vi "Save Data.vi"(8 "error in (no error)":errorcluster, 10 "signal out":waveform(dbl), 11 "Txt in":refnum<class "Txt.lvclass">) -> (0 "error out":errorcluster, 3 "Txt out":refnum<class "Txt.lvclass">)   [LabVIEW 2020, in "Txt.lvlib" / "Txt.lvclass"]
uses:
  Txt.lvclass
  Txt.lvclass/Txt.ctl
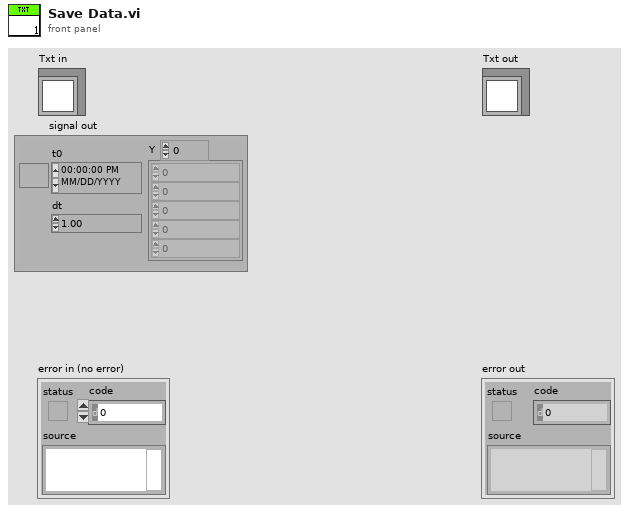
[diagram p1: front panel]
types:
  T1 = enum16{"open", "replace", "create", "open or create", "replace or create", "replace or create with confirmation"}
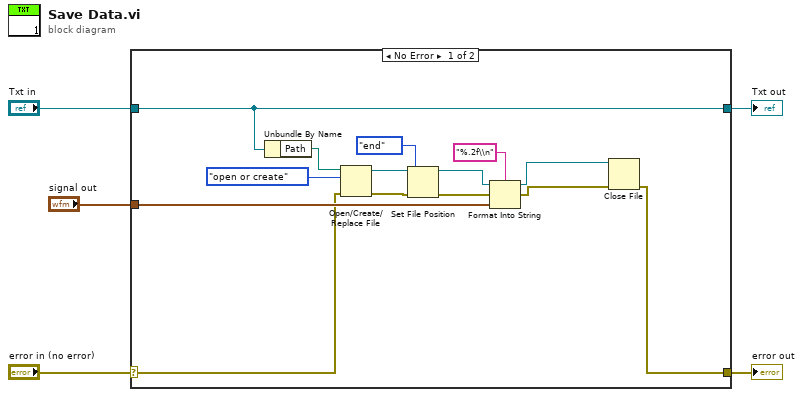
[diagram p0: block diagram]
diagram:
  n1 = case shown="No Error" "error in (no error)" {
    selector: "error in (no error)" -> [w7 w21]
    tunnel: [w6 w21] -> w4
    tunnel: [w9 w20] -> w2
    tunnel: "Txt in" -> [w9 w20]
    tunnel: "signal out" -> [w8 _]
    frame No Error {
      n2 = Unbundle By Name(w9) -> ("Path"=w19:path)
      n3 = Open/Create/Replace File(file path (use dialog)=w19, error in=w7, operation (0:open)=T1."open or create") -> (refnum out=w17:refnum<file>, error out=w16:errorcluster)  [unwired: 3 in, 1 out]
      n4 = Set File Position(refnum=w17, from (0:start)=enum16{"start", "end", "current"}."end", error in=w16) -> (refnum out=w14:refnum<file>, error out=w13:errorcluster)  [unwired: 1 in]
      n5 = Format Into String(format string="%.2f\\n", initial string=w14, error in=w13, w8) -> (resulting string=w11:refnum<file>, error out=w12:errorcluster)
      n6 = Close File(refnum=w11, error in=w12) -> (error out=w6:errorcluster)  [unwired: 1 out]
    }
    frame Error {
    }
  }
  "error out" <- w4
  "Txt out" <- w2
